vi "ApplicationRef.vi"(10 "machine name(IP)":string="127.0.0.1", 11 "port number(3363)":u16=3363) -> (0 "error out":errorcluster, 3 "Application out":refnum<vi>)   [LabVIEW 2020]
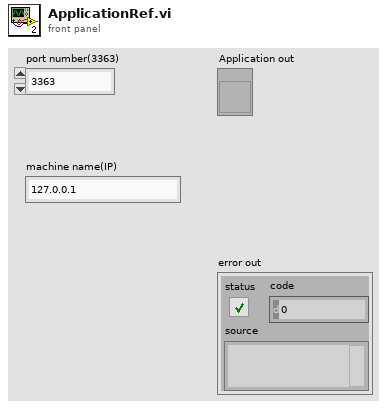
[diagram p1: front panel]
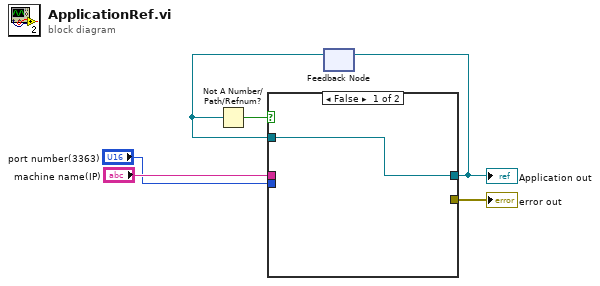
[diagram p0: block diagram]
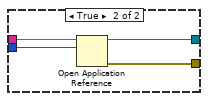
[diagram p2: hidden frame]
diagram:
  n1 = feedback #1() -> (w1:refnum<vi>)  [unwired: 1 in]
  n2 = Not A Number/Path/Refnum?(number/path/refnum=w1) -> (NaN/Path/Refnum?=w2:bool)
  n3 = case shown="False" w2 {
    tunnel: "machine name(IP)" -> [_ w11]
    tunnel: "port number(3363)" -> [_ w10]
    tunnel: [_ w9] -> w4
    tunnel: [w7 w8] -> w3
    tunnel: w1 -> [w7 _]
    frame False {
    }
    frame True {
      n4 = Open Application Reference(10:w10, 11:w11) -> (0:w9:errorcluster, 3:w8:refnum<vi>)  [unwired: 2 in]
    }
  }
  "error out" <- w4
  "Application out" <- w3
  n5 = feedback-in #1(w3) -> ()
